vi "PH_PowerUnit_BaseClass.PC_Timing Instance Status.vi"(0 "i ref in":refnum<vi>, 3 "Status":T1 items=["no info", "off/false/out", "on/true/in", "Failure", "Alarm", "Status 1", "Status 2", "Status 3"], 4 "not linked?":bool, 5 "error in (no error)":errorcluster) -> (14 "i ref out":refnum<vi>, 19 "error out":errorcluster)   [LabVIEW 2014, in "PH_PowerUnit_BaseClass.lvlib"]
doc: "This VI writes the status of the related device to own attributes."
uses:
  PH_PowerUnit_BaseClass.lvlib
  PH_StatusHandler/PH_StatusHandler.Status.ctl
  PH_Common/PH_Common.lvlib
  PH_StatusHandler/PH_StatusHandler.lvlib
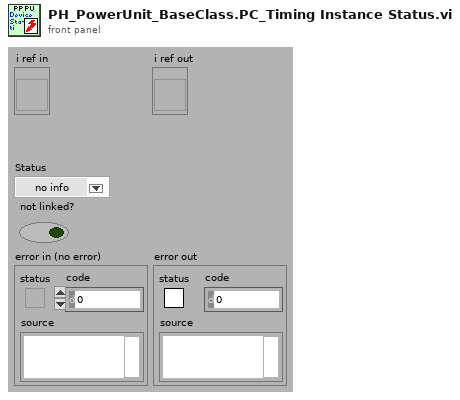
[diagram p1: front panel]
types:
  T1 = typedef "PH_StatusHandler.lvlib/PH_StatusHandler.Status.ctl" = i16
  T2 = typedef "PH_PowerUnit_BaseClass.lvlib/PH_PowerUnit_BaseClass.i attribute.ctl" = cluster{"Constructor finished":bool, "PU":cluster{"In use":bool, "Service ID in use":i32, "GUI Ref":refnum<vi>}, "Enabling":cluster{"State":T3, "GUI Ref":refnum<vi>}, "Timing":cluster{"Last Shot":dbl, "Time between Shots [Sec]":dbl, "Waiting Time over?":bool, "Service ID Waiting Time":i32, "GUI Ref":refnum<vi>, "Instance":cluster{"Status":T1, "linked?":bool, "GUI Ref":refnum<vi>}}, "Sequencer":cluster{"SM State":string, "GUI Ref":refnum<vi>, "linked":bool}, "Subscribed Trendmssgs":cluster{"Tagname":string, "Status":T1, "linked?":bool, "Shot Condition":T1, "GUI Ref":refnum<vi>}[], "PP PU":T4, "Default Voltage (V)":dbl, "GUI Refs":T5, "PSDB data":cluster{"Shot Voltage [V]":dbl, "State TO SM":T6, "Write 2 early":bool}, "State TO SM":T6}
  T3 = typedef "PH_SystemInformation.lvlib/PH_SystemInformationEnabling State.ctl" = i32
  T4 = typedef "PH_PP_Common.lvlib/PH_PP_Common.PUs.ctl" = enum16{"no Info", "PA-19mm-1", "PA-19mm-2", "PA-45mm-PILC", "PA-45mm-MAIN", "MA-PU-1", "MA-PU-2", "MA-PU-3", "MA-PU-4", "MA-PU-5", "MA-PU-6", "MA-FR", "MA-PILC", "PA-45mm-DP"}
  T5 = typedef "PH_PowerUnit_BaseClass.lvlib/PH_PowerUnit_BaseClass.GUI Refs.ctl" = cluster{"Delete Inst":refnum<vi>, "State TO SM":refnum<vi>, "State SM":refnum<vi>, "Fire":refnum<vi>}
  T6 = typedef "PH_PowerUnit_BaseClass.lvlib/PH_PowerUnit_BaseClass.SM States.ctl" = enum16{".", "Stand by", "Switch PU on", "Configure", "Set Default Voltage", "Set STANDBY", "Set READY", "Wait for Shot Cmd", "Open Dump Rods", "Open Ross Relais", "Close Ross Relais", "Switch PSU on", "Switch PSU off", "Charge", "Switch GD Channel on", "Close Dump Rods", "Rods-TO", "RR-TO", "PSU-TO", "Trigger-TO"}
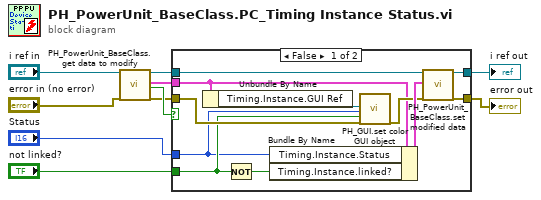
[diagram p0: block diagram]
diagram:
  n1 = call "PH_PowerUnit_BaseClass.get data to modify.vi"("i ref in"="i ref in", "error in (no error)"="error in (no error)") -> ("i ref out"=w2:refnum<vi>, "i attribute"=w1:T2, "timed out"=w4:bool, "error out"=w3:errorcluster)  [unwired: 14 in]
  n2 = case shown="False" w4 {
    tunnel: w2 -> [w21 w23]
    tunnel: [w18 w23] -> w9
    tunnel: w3 -> [w17 w22]
    tunnel: [w19 w22] -> w10
    tunnel: w1 -> [w12 _]
    tunnel: "Status" -> [w13 _]
    tunnel: "not linked?" -> [w15 _]
    frame False {
      n3 = Unbundle By Name(w12) -> ("Timing.Instance.GUI Ref"=w11:refnum<vi>)
      n4 = Not(x=w15) -> (.not. x?=w14:bool)
      n5 = Bundle By Name(cluster=w12, "Timing.Instance.Status"=w13, "Timing.Instance.linked?"=w14) -> (w20:T2)
      n6 = call "PH_GUI.set color GUI object.vi"("GUI object Ref"=w11, "State"=w13, "Blinking? (false)"=w15, "error in (no error)"=w17) -> ("error out"=w16:errorcluster)  [unwired: 15 in]
      n7 = call "PH_PowerUnit_BaseClass.set modified data.vi"("i ref in"=w21, "i attribute"=w20, "error in (no error)"=w16) -> ("i ref out"=w18:refnum<vi>, "error out"=w19:errorcluster)  [unwired: 15 in]
    }
    frame True {
    }
  }
  "error out" <- w10
  "i ref out" <- w9
